vi "SPI Transaction Timer.vi"(10 "Minimum Loop Rate (Ticks)":u32, 11 "Desired Loop Time (Ticks)":u32) -> (3 "Actual Time (Ticks)":u32)   [LabVIEW 2015, in "SPI API.lvlib"]
doc: "This VI allows the loop period to be set to a certain frequency when queuing commands to the SPI Engine. This effectively acts as a \"sample clock\" for the transactions occurring on the SPI bus, and can be used to sample SPI-based ADCs or DACs at a desired frequency."
uses:
  SPI API.lvlib
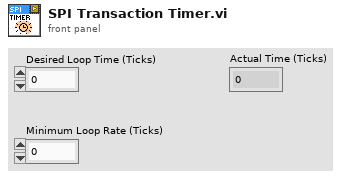
[diagram p1: front panel]
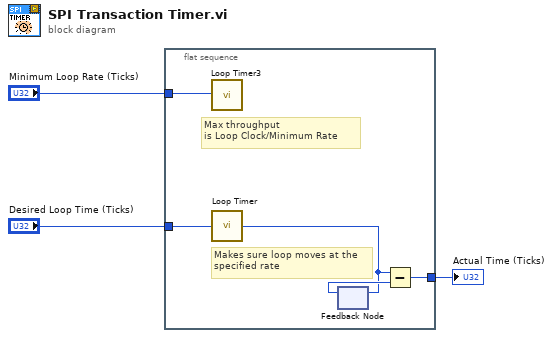
[diagram p0: block diagram]
diagram:
  n1 = flat-sequence {
    tunnel: "Desired Loop Time (Ticks)" -> [w8]
    tunnel: [w5] -> w3
    tunnel: "Minimum Loop Rate (Ticks)" -> [w4]
    frame #0 {
      # "Max throughput\nis Loop Clock/Minimum Rate"
      # "Makes sure loop moves at the\nspecified rate"
      n2 = call "Loop Timer3"("Count(Ticks)"=w4) -> ()  [unwired: 1 out]
      n3 = call "Loop Timer"("Count(Ticks)"=w8) -> ("Tick Count(Ticks)"=w6:u32)
      n4 = feedback-in #1(w6) -> ()
      n5 = feedback #1() -> (w7:u32)  [unwired: 1 out]
      n6 = Subtract(x=w6, y=w7) -> (x-y=w5:u32)
    }
  }
  "Actual Time (Ticks)" <- w3
